vi "ColorTable.vi"(11 "色码表":u32[](array[colorbox])=[16860, 5898160, 6745856, 16765184, 16711680]) -> (3 "数组":u32[](array[numeric]))   [LabVIEW 2011]
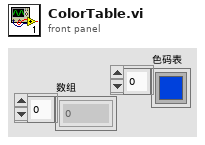
[diagram p1: front panel]
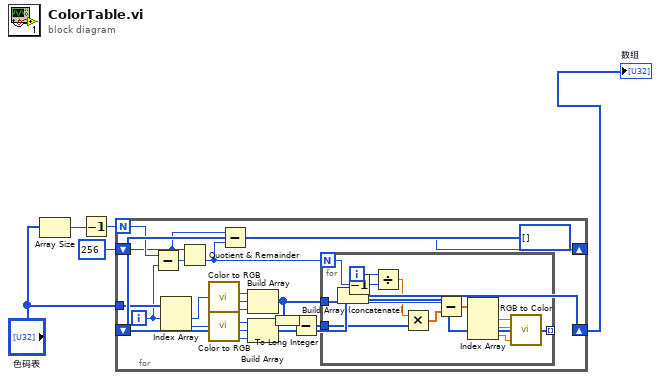
[diagram p0: block diagram]
diagram:
  n1 = Array Size(array="色码表") -> (size(s)=w3:i32)
  n2 = Decrement(x=w3) -> (x-1=w2:i32)
  n3 = for {
    N: w2 -> [w27]
    tunnel: "色码表" -> [w28]
    shift-right: [w25] -> _
    shift-left: 256 -> [w26]
    shift-right: [w7] -> w5
    shift-left: u32[] [] -> [w8]
    i -> [w23]
    n4 = Subtract(x=w27, y=w23) -> (x-y=w24:i32)
    n5 = Index Array(array=w28, index #1=w23) -> (element #1=w21:u32, element #2=w20:u32)  [unwired: 1 in]
    n6 = Quotient & Remainder(x=w26, y=w24) -> (floor(x/y)=w22:i32)  [unwired: 1 out]
    n7 = call <vilib>:"Color to RGB.vi"("Color"=w21) -> ("R"=w19:u8, "G"=w18:u8, "B"=w17:u8)  [unwired: 1 out]
    n8 = call <vilib>:"Color to RGB.vi"("Color"=w20) -> ("R"=w14:u8, "G"=w15:u8, "B"=w16:u8)  [unwired: 1 out]
    n9 = Subtract(x=w26, y=w22) -> (x-y=w25:i32)
    n10 = Build Array(w19, w18, w17) -> (w11:u8[])
    n11 = Build Array(w14, w15, w16) -> (w13:u8[])
    n12 = To Long Integer(number=w11) -> (32bit integer=w9:i32[])
    n13 = Subtract(x=w9, y=w13) -> (x-y=w12:i32[])
    n14 = for {
      N: w22 -> [w40]
      tunnel: w12 -> [w35]
      tunnel: w11 -> [w37]
      tunnel: [w29] -> w10 mode=indexing
      i -> [w38]
      n15 = Decrement(x=w40) -> (x-1=w39:i32)
      n16 = Divide(x=w38, y=w39) -> (x/y=w36:dbl)
      n17 = Multiply(x=w36, y=w35) -> (x*y=w34:dbl[])
      n18 = Subtract(x=w37, y=w34) -> (x-y=w33:dbl[])
      n19 = Index Array(array=w33) -> (element #1=w32:dbl, element #2=w31:dbl, element #3=w30:dbl)  [unwired: 3 in]
      n20 = call <vilib>:"RGB to Color.vi"("B"=w30, "G"=w31, "R"=w32) -> ("Color"=w29:u32)
    }
    n21 = Build Array (concatenate)(w8, w10) -> (w7:u32[])
  }
  "数组" <- w5
